vi "_Fit VI window to Visible Content.vi"(4 "error in (no error)":errorcluster, 6 "border spacing (2 px)":i32=2, 7 "VI Ref (calling VI)":refnum<vi>) -> (0 "error out":errorcluster, 3 "dup VI Ref":refnum<vi>)   [LabVIEW 2017]
doc: "This utility will fit (resize and center) a VI (defined by the \"VI Ref\" input) about the all of the Front Panel object. It will add a border defined by border spacing in units of pixels. If no VI Reference is passed in, it will operate on the calling VI."
panel:
  # "Fit VI window to Content.vi\n\nFits a VI's front panel window to its FP Contents.\n\nPlease visit http://www.OpenG.org to learn about the\nOpen Source LabVIEW software movement.\n\nNOTICE -- YOU MUST LEAVE THIS NOTICE IN PLACE.  PER THE TERMS OF THE LICENSE BELOW, YOU MAY SUBLICENSE THIS SOFTWARE \nIN ANY WAY THAT DOES NOT CONFLICT WITH THIS LICENSE.\n\n### BSD License (http://www.opensource.org/licenses/bsd-license.php) Begin ###\n \nCopyright (c) 2002-2004, Jim Kring <jim@jimkring.com>\nCopyright (c) 2002, Cal-Bay Systems, Inc. <info@calbay.com>\n\nAll rights reserved.\n\nRedistribution and use in source and binary forms, with or without modification, are permitted provided that the following conditions are met:\n\n    * Redistributions of source code must retain the above copyright notice, this list of conditions and the following disclaimer.\n    * Redistributions in binary form must reproduce the above copyright notice, this list of conditions and the following disclaimer in the \n       documentation and/or other materials provided with the distribution.\n    * Neither the name of SciWare, James Kring, Inc., nor the names of its contributors may be used to endorse or promote products derived \n       from this software without specific prior written permission.\n\nTHIS SOFTWARE IS PROVIDED BY THE COPYRIGHT HOLDERS AND CONTRIBUTORS \"AS IS\" AND ANY EXPRESS OR IMPLIED WARRANTIES, \nINCLUDING, BUT NOT LIMITED TO, THE IMPLIED WARRANTIES OF MERCHANTABILITY AND FITNESS FOR A PARTICULAR PURPOSE ARE \nDISCLAIMED. IN NO EVENT SHALL THE COPYRIGHT OWNER OR CONTRIBUTORS BE LIABLE FOR ANY DIRECT, INDIRECT, INCIDENTAL,\n SPECIAL, EXEMPLARY, OR CONSEQUENTIAL DAMAGES (INCLUDING, BUT NOT LIMITED TO, PROCUREMENT OF SUBSTITUTE GOODS OR \nSERVICES; LOSS OF USE, DATA, OR PROFITS; OR BUSINESS INTERRUPTION) HOWEVER CAUSED AND ON ANY THEORY OF LIABILITY, \nWHETHER IN CONTRACT, STRICT LIABILITY, OR TORT (INCLUDING NEGLIGENCE OR OTHERWISE) ARISING IN ANY WAY OUT OF THE USE \nOF THIS SOFTWARE, EVEN IF ADVISED OF THE POSSIBILITY OF SUCH DAMAGE.\n\n### BSD License End ###"
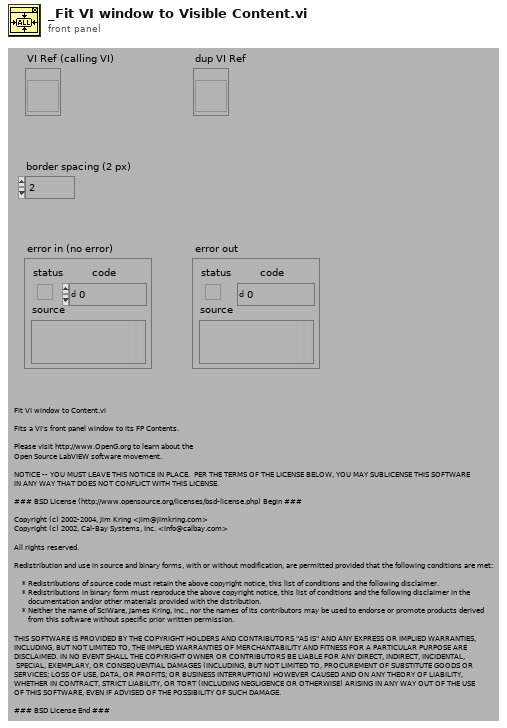
[diagram p1: front panel]
types:
  T1 = typedef "LVRectTypeDef.ctl" = cluster{"Left":i16, "Top":i16, "Right":i16, "Bottom":i16}
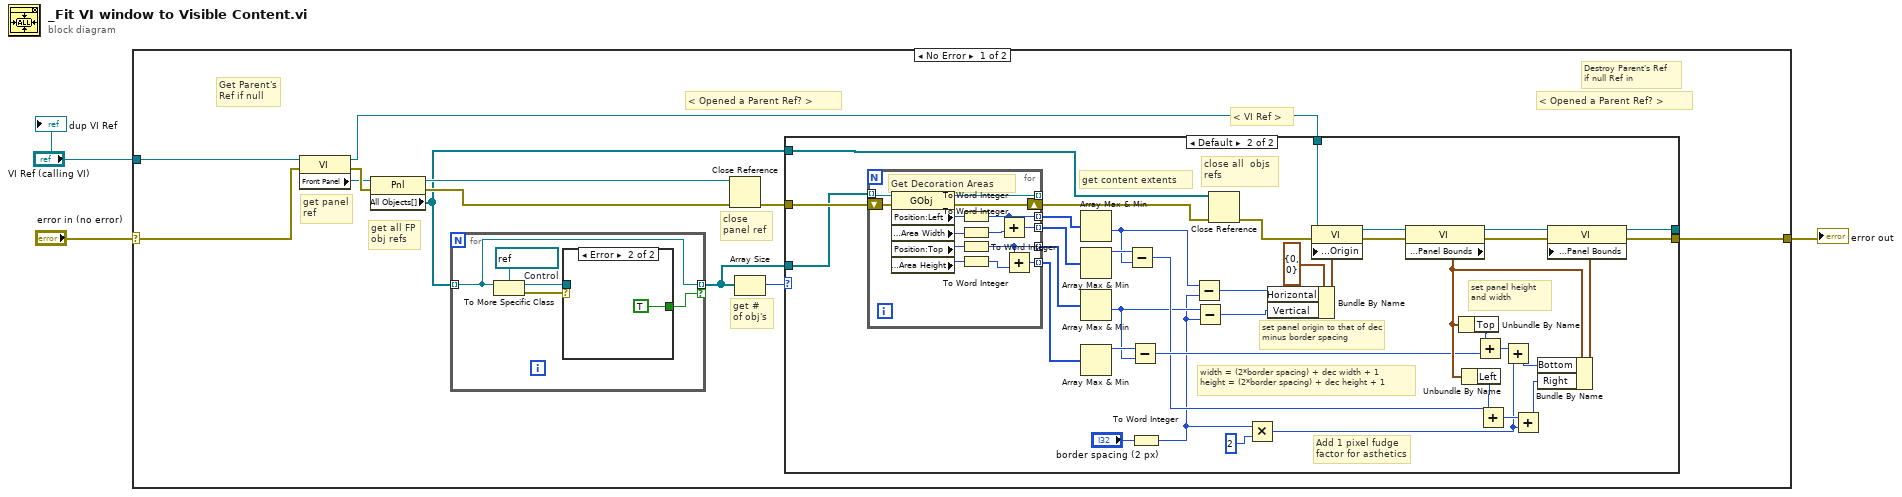
[diagram p0: block diagram]
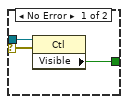
[diagram p2: hidden frame]
diagram:
  n1 = case shown="No Error" "error in (no error)" {
    selector: "error in (no error)" -> [w6 w79]
    tunnel: [w9 w79] -> w3
    tunnel: "VI Ref (calling VI)" -> [w7 _]
    frame No Error {
      # "< Opened a Parent Ref? >"
      # "< Opened a Parent Ref? >"
      # "Destroy Parent's Ref\nif null Ref in"
      # "Get Parent's\nRef if null"
      # "get # of obj's"
      # "get panel ref"
      # "get all FP obj refs"
      # "close panel ref"
      # "< VI Ref >"
      n2 = property on="Property Node" class="VI"(reference=w7, error in=w6) -> (reference out=w15:refnum<vi>, error out=w13:errorcluster, "Front Panel"=w11:refnum<vi>)
      n3 = property on="Property Node" class="Pnl"(reference=w11, error in=w13) -> (reference out=w14:refnum<vi>, error out=w12:errorcluster, "All Objects[]"=w5:refnum<vi>[])
      n4 = for {
        tunnel: [w16] -> w4 mode=indexing if=w17
        tunnel: w5 -> [w16] mode=indexing
        w19 = refnum<vi> refnum  # Control
        n5 = To More Specific Class(target class=w19, reference=w16) -> (specific class reference=w20:refnum<vi>, error out=w18:errorcluster)  [unwired: 1 in]
        n6 = case shown="Error" w18 {
          selector: w18 -> [w22 _]
          tunnel: w20 -> [w23 _]
          tunnel: [w21 TRUE ("Visible")] -> w17
          frame No Error {
            n7 = property class="Ctl"(reference=w23, error in=w22) -> ("Visible"=w21:bool)  [unwired: 2 out]
          }
          frame Error {
          }
        }
      }
      n8 = Close Reference(reference=w14, error in (no error)=w12) -> (error out=w10:errorcluster)
      n9 = Array Size(array=w4) -> (size(s)=w8:i32)
      n10 = case shown="Default" w8 {
        tunnel: w15 -> [w26 w62]
        tunnel: w10 -> [w25 w49]
        tunnel: [w25 w44] -> w9
        tunnel: [w26 w43] -> _
        tunnel: w5 -> [_ w28]
        tunnel: w4 -> [_ w27]
        frame 0 {
          # "do nothing if no objects"
        }
        frame Default {
          # "width = (2*border spacing) + dec width + 1\nheight = (2*border spacing) + dec height + 1"
          # "set panel height and width"
          # "set panel origin to that of dec minus border spacing"
          # "close all  objs refs"
          # "get content extents"
          # "Add 1 pixel fudge factor for asthetics"
          n11 = for {
            tunnel: w27 -> [w78] mode=indexing
            shift-right: [w76] -> w31
            shift-left: w49 -> [w77]
            tunnel: [w75] -> _ mode=indexing
            tunnel: [w71] -> w41 mode=indexing
            tunnel: [w73] -> w40 mode=indexing
            tunnel: [w67] -> w39 mode=indexing
            tunnel: [w72] -> w38 mode=indexing
            # "Get Decoration Areas"
            n12 = property class="GObj"(reference=w78, error in=w77) -> (reference out=w75:refnum<vi>, error out=w76:errorcluster, "Position:Left"=w74:i32, "Bounds:Area Width"=w70:u32, "Position:Top"=w68:i32, "Bounds:Area Height"=w66:u32)
            n13 = To Word Integer(number=w74) -> (16bit integer=w71:i16)
            n14 = To Word Integer(number=w70) -> (16bit integer=w69:i16)
            n15 = To Word Integer(number=w68) -> (16bit integer=w67:i16)
            n16 = To Word Integer(number=w66) -> (16bit integer=w65:i16)
            n17 = Add(x=w71, y=w69) -> (x+y=w73:i16)
            n18 = Add(x=w67, y=w65) -> (x+y=w72:i16)
          }
          n19 = Array Max & Min(array=w41) -> (min value=w32:i16)  [unwired: 3 out]
          n20 = Array Max & Min(array=w40) -> (max value=w35:i16)  [unwired: 3 out]
          n21 = Array Max & Min(array=w39) -> (min value=w33:i16)  [unwired: 3 out]
          n22 = Array Max & Min(array=w38) -> (max value=w37:i16)  [unwired: 3 out]
          n23 = Subtract(x=w35, y=w32) -> (x-y=w34:i16)
          n24 = Subtract(x=w37, y=w33) -> (x-y=w36:i16)
          n25 = To Word Integer(number="border spacing (2 px)") -> (16bit integer=w29:i16)
          n26 = Subtract(x=w32, y=w29) -> (x-y=w52:i16)
          n27 = Subtract(x=w33, y=w29) -> (x-y=w53:i16)
          n28 = Close Reference(reference=w28, error in (no error)=w31) -> (error out=w30:errorcluster)
          n29 = Multiply(x=w29, y=i16 2) -> (x*y=w42:i16)
          n30 = Bundle By Name(cluster=cluster{"Horizontal":i16, "Vertical":i16} {"Horizontal"=0, "Vertical"=0} ("Front Panel Window:Origin"), "Horizontal"=w52, "Vertical"=w53) -> (w50:cluster{"Horizontal":i16, "Vertical":i16})
          n31 = property on="Property Node" class="VI"(reference=w62, error in=w30, "Front Panel Window:Origin"=w50) -> (reference out=w63:refnum<vi>, error out=w46:errorcluster)
          n32 = property on="Property Node" class="VI"(reference=w63, error in=w46) -> (reference out=w64:refnum<vi>, error out=w45:errorcluster, "Front Panel Window:Panel Bounds"=w54:T1)
          n33 = Unbundle By Name(w54) -> ("Top"=w55:i16)
          n34 = Unbundle By Name(w54) -> ("Left"=w56:i16)
          n35 = Add(x=w55, y=w36) -> (x+y=w60:i16)
          n36 = Add(x=w56, y=w34) -> (x+y=w58:i16)
          n37 = Add(x=w60, y=w42) -> (x+y=w61:i16)
          n38 = Add(x=w58, y=w42) -> (x+y=w59:i16)
          n39 = Bundle By Name(cluster=w54, "Bottom"=w61, "Right"=w59) -> (w57:T1)
          n40 = property on="Property Node" class="VI"(reference=w64, error in=w45, "Front Panel Window:Panel Bounds"=w57) -> (reference out=w43:refnum<vi>, error out=w44:errorcluster)
        }
      }
    }
    frame Error {
    }
  }
  "error out" <- w3
  "dup VI Ref" <- "VI Ref (calling VI)"
